vi "ProcessSerialUpdates.vi"(11 "MockDisplacementSettings":T1={"SerialPort"="Slot3\\Port1", "BufferUpdateFIFO"="MockDisplacementCommandFIFO", "DisplacementMemory"="DisplacementMemory"}) -> ()   [LabVIEW 2016, in "FPGAMockDisplacement.lvlib"]
uses:
  FPGAMockDisplacement.lvlib
  DataTypes/MockDisplacementSettings.ctl
  <vilib>/rvi/Emulation/niFpgaGetClockAttributes.vi
  <vilib>/rvi/Emulation/niFpgaSctlEmulationGetInTimedLoop.vi
  <vilib>/rvi/Emulation/niFpgaEmulationReportErrorSimple.vi
  <vilib>/rvi/eio/common/nirviEmuTemplateMethod_errors.vi
  <vilib>/rvi/DataTransferAndStorage/Container/Common/niFpgaContainerExecOnDevCompGetState.vi
  <vilib>/rvi/Emulation/niFpgaEmulationIsFPGAContextNoSignature.vi
  <vilib>/rvi/DataTransferAndStorage/Container/Common/niFpgaContainerGetUniqueNameForEmu.vi
  <vilib>/rvi/Emulation/niFpgaProcessEmulError.vi
  <vilib>/rvi/errors/nirviReportUnexpectedCaseInternalError (U32).vi
  <vilib>/rvi/Memory/Memory_Emulation/niFpgaMemoryEmulationCacheClearOnFirstRun.vi
  <vilib>/rvi/Memory/Memory_Emulation/nirvimemoryEmulationManagerCache_MakeExclusive.vi
  <vilib>/rvi/Memory/Memory_Emulation/niFpgaMemoryEmulationValidateCache.vi
  <vilib>/rvi/Memory/Memory_Emulation/nirvimemoryEmulationManagerCache_InsertValue.vi
  <vilib>/Utility/error.llb/Clear Errors.vi
  <vilib>/rvi/Memory/Memory_Emulation/nirvimemoryEmulationManagerCache_ReleaseExclusive.vi
  <vilib>/rvi/Memory/Memory_Emulation/nirvimemoryEmulationManagerCache_GetValue.vi
  <vilib>/rvi/Memory/Memory_Emulation/nirvimemoryEmulationManagerCache_SetValue.vi
  <vilib>/rvi/Emulation/niFpgaSctlEmulationResourceMgr.vi
  <vilib>/rvi/Emulation/niFpgaCriticalErrorInLSC.vi
  <vilib>/eio/EIOMethodNode/EIOMethodNode.xnode
  <vilib>/rvi/DataTransferAndStorage/Container/XNode/niFpgaContainer.xnode
  <vilib>/rvi/Memory/Memory_Emulation/niFpgaMemoryEmulationRefIn.vi
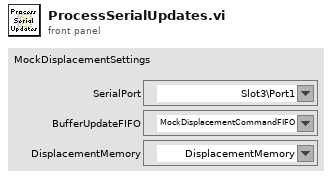
[diagram p1: front panel]
types:
  T1 = typedef "FPGAMockDisplacement.lvlib/MockDisplacementSettings.ctl" = cluster{"SerialPort":refnum<k21>, "BufferUpdateFIFO":refnum<k21>, "DisplacementMemory":refnum<k21>}
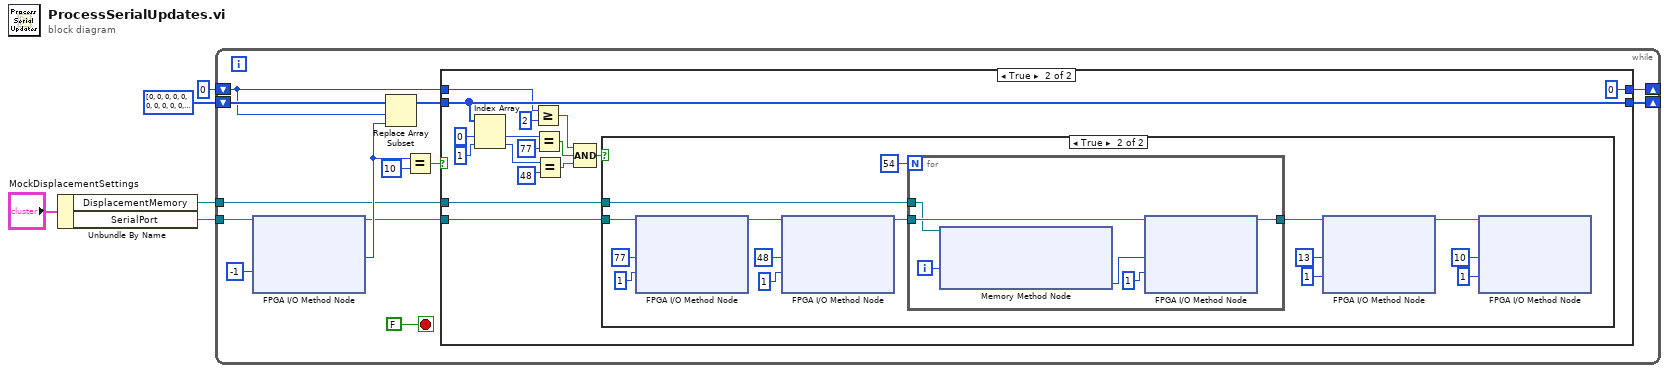
[diagram p0: block diagram]
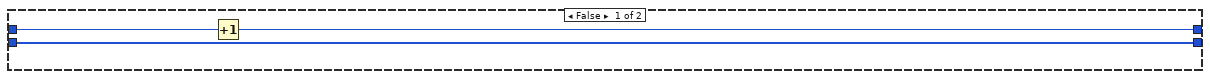
[diagram p2: hidden frame]
diagram:
  n1 = Unbundle By Name("MockDisplacementSettings") -> ("DisplacementMemory"=w1:refnum<k21>, "SerialPort"=w2:refnum<k21>)
  n2 = while {
    tunnel: w2 -> [w18]
    shift-right: [w10] -> _
    shift-left: u8[] [0, 0, 0, 0, 0, 0, 0, 0, 0, 0, 0, 0, 0, 0, 0, 0, 0, 0, 0, 0, 0, 0, 0, 0, 0, 0, 0, 0, 0, 0, 0, 0, 0, 0, 0, 0, 0, 0, 0, 0, 0, 0, 0, 0, 0, 0, 0, 0, 0, 0, 0, 0, 0, 0, 0, 0, 0, 0, 0, 0, 0, 0, 0, 0, 0, 0, 0, 0, 0, 0, 0, 0, 0, 0, 0, 0, 0, 0, 0, 0, 0, 0, 0, 0, 0, 0, 0, 0, 0, 0, 0, 0, 0, 0, 0, 0, 0, 0, 0, 0, 0, 0, 0, 0, 0, 0, 0, 0, 0, 0, 0, 0, 0, 0, 0, 0, 0, 0, 0, 0, 0, 0, 0, 0, 0, 0, 0, 0, 0, 0, 0, 0, 0, 0, 0, 0, 0, 0, 0, 0, 0, 0, 0, 0, 0, 0, 0, 0, 0, 0, 0, 0, 0, 0, 0, 0, 0, 0, 0, 0, 0, 0, 0, 0, 0, 0, 0, 0, 0, 0, 0, 0, 0, 0, 0, 0, 0, 0, 0, 0, 0, 0, 0, 0, 0, 0, 0, 0, 0, 0, 0, 0, 0, 0, 0, 0, 0, 0, 0, 0, 0, 0, 0, 0, 0, 0, 0, 0, 0, 0, 0, 0, 0, 0, 0, 0, 0, 0, 0, 0, 0, 0, 0, 0, 0, 0, 0, 0, 0, 0, 0, 0, 0, 0, 0, 0, 0, 0, 0, 0, 0, 0, 0, 0, 0, 0, 0, 0, 0, 0, 0, 0, 0, 0, 0, 0] -> [w15]
    shift-right: [w11] -> _
    shift-left: i16 0 -> [w7]
    tunnel: w1 -> [w8]
    stop <- FALSE stop-if-true
    n3 = xnode "FPGA I/O Method Node"("FPGA I/O In"=w18, "Timeout (ms)"=-1) -> ("FPGA I/O Out"=w9:refnum<k21>, "Data"=w14:u8)  [unwired: 1 out]
    n4 = Replace Array Subset(array=w15, new element=w14, index=w7) -> (w12:u8[])
    n5 = Equal?(x=w14, y=u8 10) -> (x = y?=w13:bool)
    n6 = case shown="True" w13 {
      tunnel: w12 -> [w21 w35]
      tunnel: [w19 i16 0] -> w11
      tunnel: w7 -> [w20 w27]
      tunnel: [w21 w35] -> w10
      tunnel: w9 -> [_ w31]
      tunnel: w8 -> [_ w29]
      frame False {
        n7 = Increment(x=w20) -> (x+1=w19:i16)
      }
      frame True {
        n8 = Index Array(array=w35, index #1=0 ("index"), index #2=1 ("index")) -> (element #1=w30:u8, element #2=w33:u8)
        n9 = Greater Or Equal?(x=w27, y=i16 2) -> (x >= y?=w24:bool)
        n10 = Equal?(x=w30, y=u8 77) -> (x = y?=w23:bool)
        n11 = Equal?(x=w33, y=u8 48) -> (x = y?=w22:bool)
        n12 = Compound Arithmetic op=AND(w24, w23, w22) -> (w25:bool)
        n13 = case shown="True" w25 {
          tunnel: w31 -> [_ w52]
          tunnel: w29 -> [_ w40]
          frame False {
          }
          frame True {
            n14 = xnode "FPGA I/O Method Node"("FPGA I/O In"=w52, "Data"=u8 77, "Timeout (ms)"=1) -> ("FPGA I/O Out"=w50:refnum<k21>)  [unwired: 1 out]
            n15 = xnode "FPGA I/O Method Node"("FPGA I/O In"=w50, "Data"=u8 48, "Timeout (ms)"=1) -> ("FPGA I/O Out"=w48:refnum<k21>)  [unwired: 1 out]
            n16 = for {
              N: 54 -> [_]
              tunnel: w48 -> [w57]
              tunnel: [w55] -> w46
              tunnel: w40 -> [w54]
              i -> [w58]
              n17 = xnode ("Memory Method Node")("Address"=w58, "Memory In"=w54) -> ("Data"=w56:u8)  [unwired: 1 out]
              n18 = xnode "FPGA I/O Method Node"("FPGA I/O In"=w57, "Data"=w56, "Timeout (ms)"=1) -> ("FPGA I/O Out"=w55:refnum<k21>)  [unwired: 1 out]
            }
            n19 = xnode "FPGA I/O Method Node"("FPGA I/O In"=w46, "Data"=u8 13, "Timeout (ms)"=1) -> ("FPGA I/O Out"=w44:refnum<k21>)  [unwired: 1 out]
            n20 = xnode "FPGA I/O Method Node"("FPGA I/O In"=w44, "Data"=u8 10, "Timeout (ms)"=1) -> ()  [unwired: 2 out]
          }
        }
      }
    }
  }
